vi "GetActorEnqueue.vi"(8 "error in (no error)":errorcluster, 10 "name":string, 11 "ActorMap in":refnum<class "ActorMap.lvclass">) -> (0 "error out":errorcluster, 1 "Enqueue":refnum<class "Message Enqueuer.lvclass">, 2 "key not found?":bool, 3 "ActorMap out":refnum<class "ActorMap.lvclass">)   [LabVIEW 2020, in "ActorMap.lvclass"]
uses:
  ActorMap.lvclass
  <vilib>/ActorFramework/Message Enqueuer/Message Enqueuer.lvclass
  ActorMap.lvclass/ActorMap.ctl
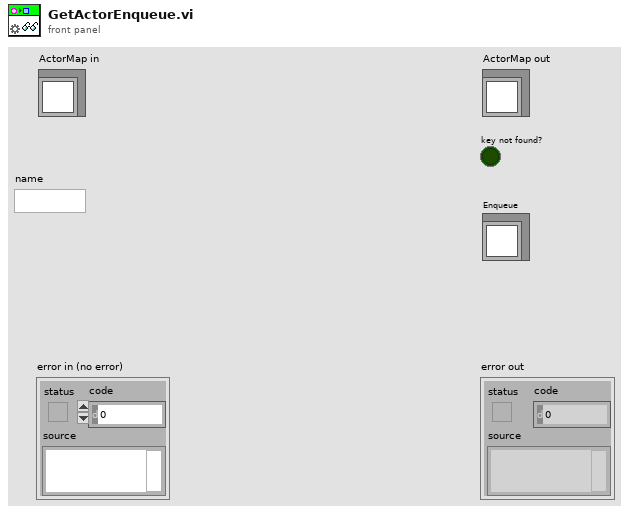
[diagram p1: front panel]
types:
  T1 = map{string, refnum<class "Message Enqueuer.lvclass">}
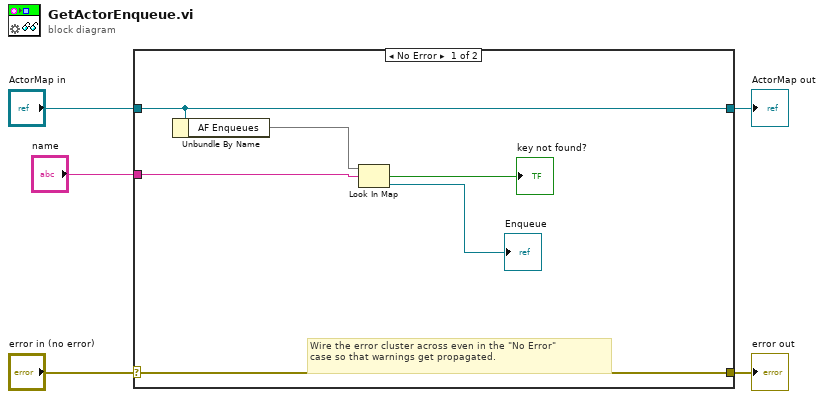
[diagram p0: block diagram]
diagram:
  n1 = case shown="No Error" "error in (no error)" {
    selector: "error in (no error)" -> [w11 w13]
    tunnel: [w11 w13] -> w4
    tunnel: [w8 w12] -> w2
    tunnel: "ActorMap in" -> [w8 w12]
    tunnel: "name" -> [w9 _]
    frame No Error {
      # "Wire the error cluster across even in the \"No Error\"\ncase so that warnings get propagated."
      n2 = Unbundle By Name(w8) -> ("AF Enqueues"=w10:T1)
      n3 = Look In Map(map=w10, key=w9) -> (key not found?=→"key not found?":bool, value=→"Enqueue":refnum<class "Message Enqueuer.lvclass">)  [unwired: 1 in]
    }
    frame Error {
    }
  }
  "error out" <- w4
  "ActorMap out" <- w2
